vi "ReceiveTCPfromPi_Binary_queue.vi"() -> ()   [LabVIEW 2014]
uses:
  <vilib>/Utility/file.llb/Write To Spreadsheet File (string).vi
  <vilib>/Utility/file.llb/Write To Spreadsheet File (DBL).vi
panel:
  in  "Description":string
  out "Binary File Refnum":refnum<file>
  in  "Record":bool
  in  "Plot 3":u16(ring) items=["gpsTimeUTC", "cT", "EKF VelN", "EKF VelE", "EKF VelD", "EKF PosN", "EKF PosE", "EKF PosD", "EKF Roll", "EKF Pitch", "EKF Yaw", "EKF Lat", "EKF Lon", "EKF Alt", "CMP VelN", "CMP VelE", "CMP VelD", "CMP PosN", "CMP PosE", "CMP PosD", "CMP Roll", "CMP Pitch", "CMP Yaw", "CMP Lat", "CMP Lon", "CMP Alt", "GPS Lat", "GPS Lon", "GPS Alt", "GPS VelN", "GPS VelE", "GPS VelD", "AccelX", "AccelY", "AccelZ", "GyroX", "GyroY", "GyroZ", "MagX", "MagY", "MagZ", "piAlpha", "piPfwd", "piP45", "ardAlpha", "ardPfwd", "ardP45", "Alpha", "Beta"]
  in  "Plot 2":u16(ring) items=["gpsTimeUTC", "cT", "EKF VelN", "EKF VelE", "EKF VelD", "EKF PosN", "EKF PosE", "EKF PosD", "EKF Roll", "EKF Pitch", "EKF Yaw", "EKF Lat", "EKF Lon", "EKF Alt", "CMP VelN", "CMP VelE", "CMP VelD", "CMP PosN", "CMP PosE", "CMP PosD", "CMP Roll", "CMP Pitch", "CMP Yaw", "CMP Lat", "CMP Lon", "CMP Alt", "GPS Lat", "GPS Lon", "GPS Alt", "GPS VelN", "GPS VelE", "GPS VelD", "AccelX", "AccelY", "AccelZ", "GyroX", "GyroY", "GyroZ", "MagX", "MagY", "MagZ", "piAlpha", "piPfwd", "piP45", "ardAlpha", "ardPfwd", "ardP45", "Alpha", "Beta"]
  in  "Plot 1":u16(ring) items=["gpsTimeUTC", "cT", "EKF VelN", "EKF VelE", "EKF VelD", "EKF PosN", "EKF PosE", "EKF PosD", "EKF Roll", "EKF Pitch", "EKF Yaw", "EKF Lat", "EKF Lon", "EKF Alt", "CMP VelN", "CMP VelE", "CMP VelD", "CMP PosN", "CMP PosE", "CMP PosD", "CMP Roll", "CMP Pitch", "CMP Yaw", "CMP Lat", "CMP Lon", "CMP Alt", "GPS Lat", "GPS Lon", "GPS Alt", "GPS VelN", "GPS VelE", "GPS VelD", "AccelX", "AccelY", "AccelZ", "GyroX", "GyroY", "GyroZ", "MagX", "MagY", "MagZ", "piAlpha", "piPfwd", "piP45", "ardAlpha", "ardPfwd", "ardP45", "Alpha", "Beta"]
  out "Num Characters Lost":i32
  out "Spreadsheet Datalog File":path=path "C:/Users/romneyj/Desktop/EKFDatalog2.txt"
  out "Binary Datalog File":path=path "C:/Users/romneyj/Desktop/EKFDatalog.txt"
  out "Chart Values":dbl[](array[numeric]) format="%#_14f"
  out "Chart":cluster{"[0]":dbl, "[1]":dbl, "[2]":dbl}(graph)
  in  "Values to Display":dbl(slide)=100.0 min=10.0 max=2000.0 step=10.0 scale=10.0..2000.0
  out "error out":errorcluster
  out "before substring":string
  in  "stop":bool
  in  "Port":u16=5005
  in  "IP Address":string="155.31.242.65"
  # "Plot Values"
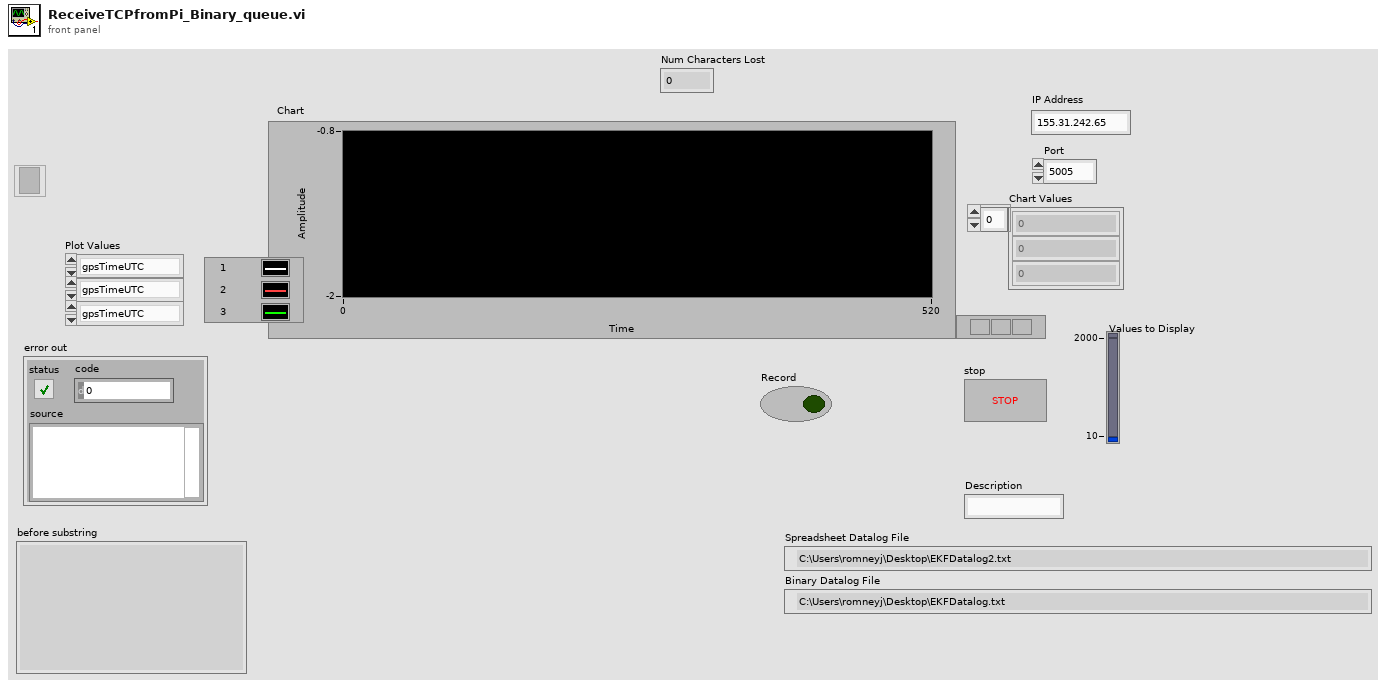
[diagram p1: front panel]
types:
  T1 = cluster{"gpsTimeUTC":i64, "cT":dbl, "EKF VelN":sgl, "EKF VelE":sgl, "EKF VelD":sgl, "EKF PosN":sgl, "EKF PosE":sgl, "EKF PosD":sgl, "EKF Roll":sgl, "EKF Pitch":sgl, "EKF Yaw":sgl, "EKF Lat":dbl, "EKF Lon":dbl, "EKF Alt":sgl, "CMP VelN":sgl, "CMP VelE":sgl, "CMP VelD":sgl, "CMP PosN":sgl, "CMP PosE":sgl, "CMP PosD":sgl, "CMP Roll":sgl, "CMP Pitch":sgl, "CMP Yaw":sgl, "CMP Lat":dbl, "CMP Lon":dbl, "CMP Alt":sgl, "GPS Lat":dbl, "GPS Lon":dbl, "GPS Alt":sgl, "GPS VelN":sgl, "GPS VelE":sgl, "GPS VelD":sgl, "AccelX":sgl, "AccelY":sgl, "AccelZ":sgl, "GyroX":sgl, "GyroY":sgl, "GyroZ":sgl, "MagX":sgl, "MagY":sgl, "MagZ":sgl, "piAlpha":sgl, "piPfwd":u16, "piP45":u16, "ardAlpha":sgl, "ardPfwd":u16, "ardP45":u16, "Alpha":sgl, "Beta":sgl}
  T2 = enum16{"open", "replace", "create", "open or create", "replace or create", "replace or create with confirmation"}
  T3 = enum16{"big-endian, network order", "native, host order", "little-endian"}
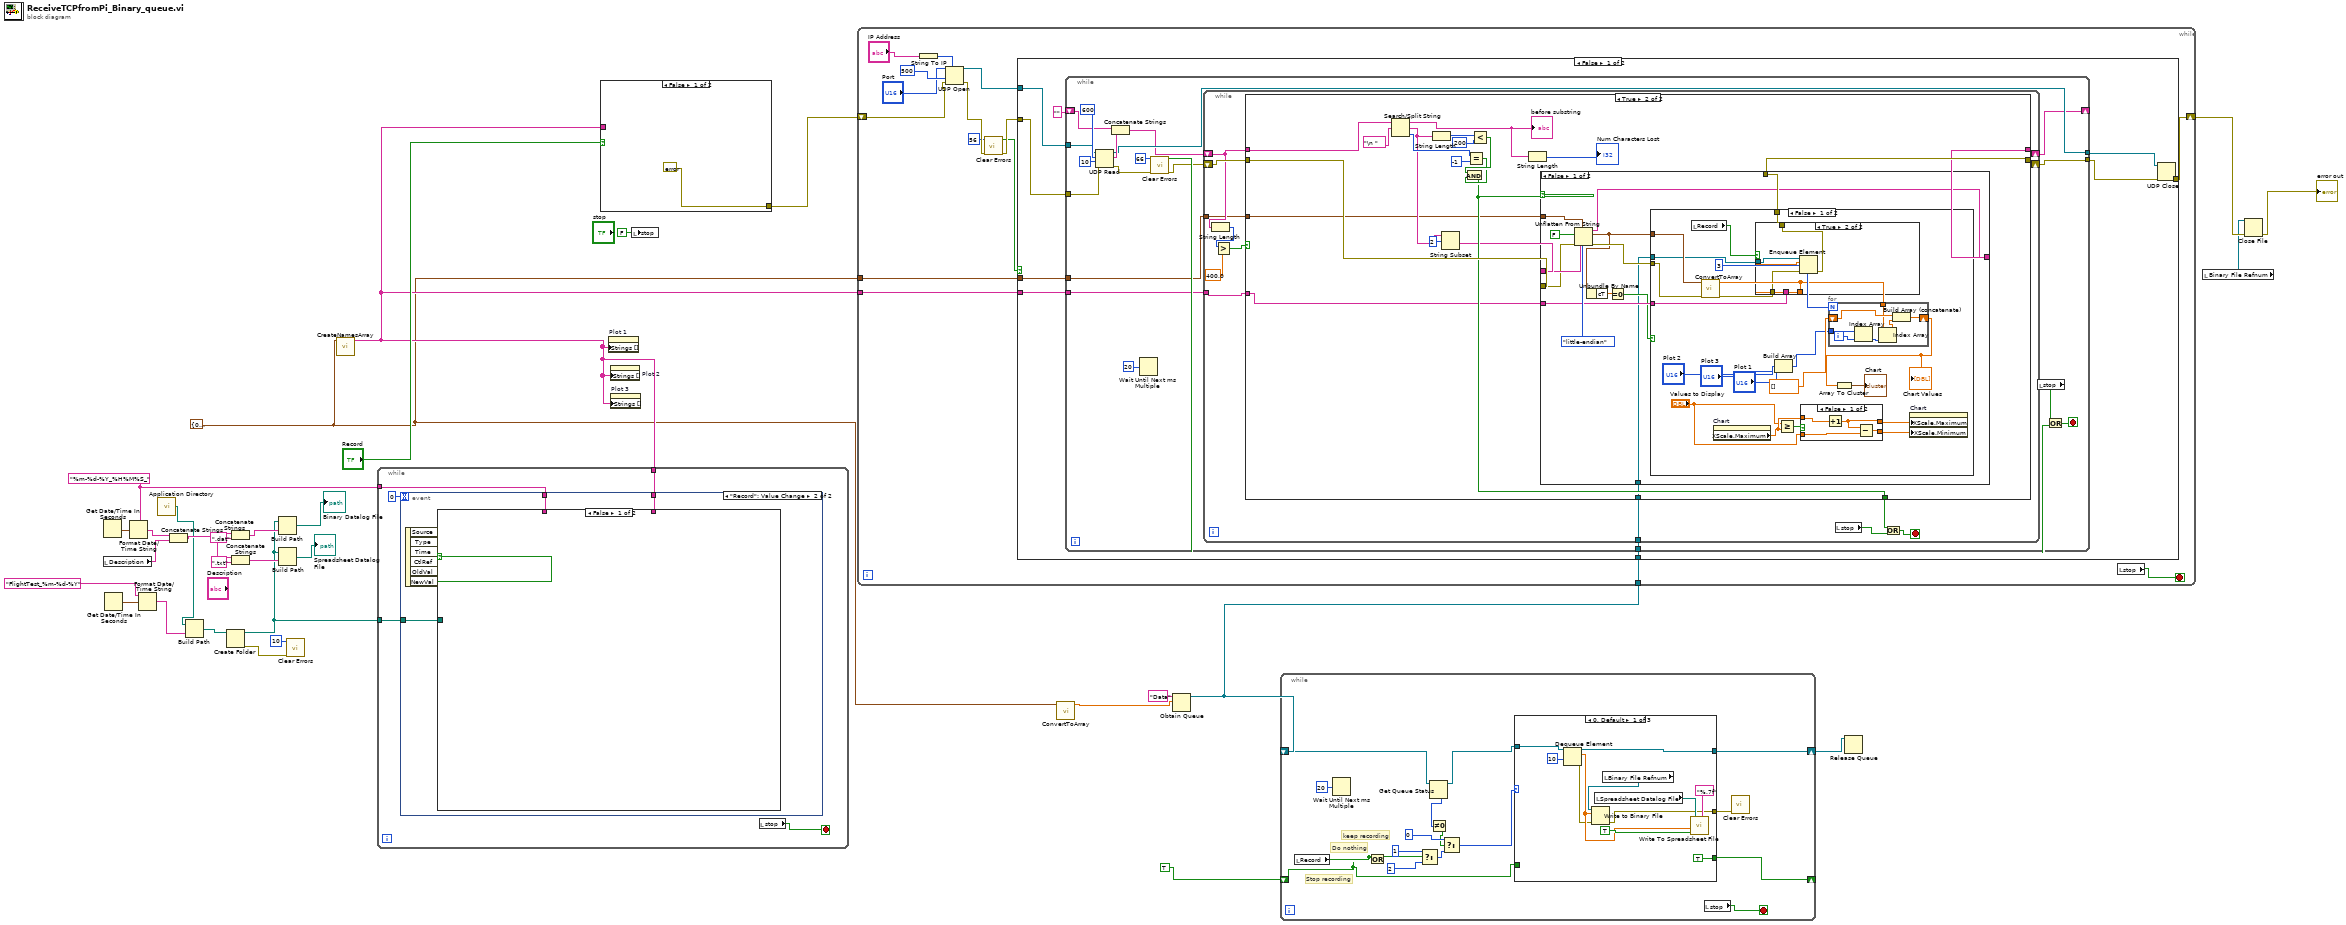
[diagram p0: block diagram]
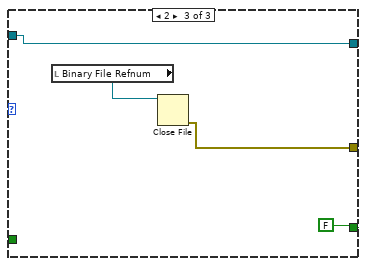
[diagram p3: hidden frame]
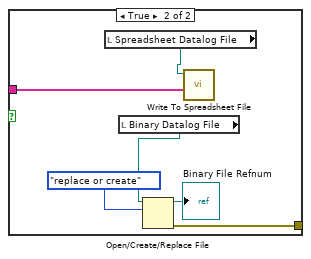
[diagram p4: hidden frame]
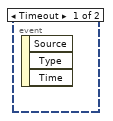
[diagram p5: hidden frame]
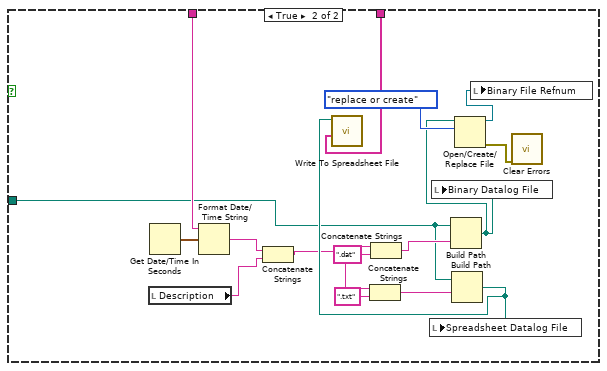
[diagram p6: hidden frame]
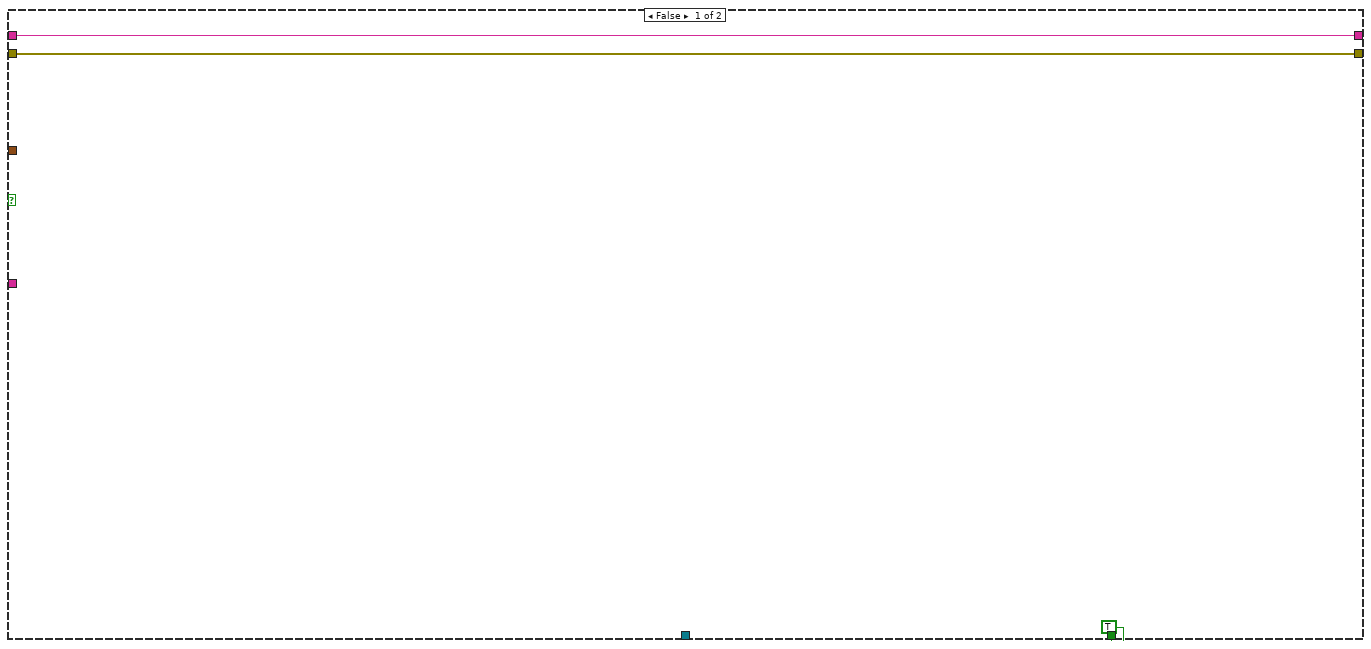
[diagram p7: hidden frame]
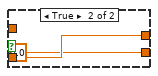
[diagram p9: hidden frame]
diagram:
  w18 = "%m-%d-%Y_%H%M%S_" ("time format string (%c)")
  w3 = T1 {"gpsTimeUTC"=0, "cT"=0.0, "EKF VelN"=0.0, "EKF VelE"=0.0, "EKF VelD"=0.0, "EKF PosN"=0.0, "EKF PosE"=0.0, "EKF PosD"=0.0, "EKF Roll"=0.0, "EKF Pitch"=0.0, "EKF Yaw"=0.0, "EKF Lat"=0.0, "EKF Lon"=0.0, "EKF Alt"=0.0, "CMP VelN"=0.0, "CMP VelE"=0.0, "CMP VelD"=0.0, "CMP PosN"=0.0, "CMP PosE"=0.0, "CMP PosD"=0.0, "CMP Roll"=0.0, "CMP Pitch"=0.0, "CMP Yaw"=0.0, "CMP Lat"=0.0, "CMP Lon"=0.0, "CMP Alt"=0.0, "GPS Lat"=0.0, "GPS Lon"=0.0, "GPS Alt"=0.0, "GPS VelN"=0.0, "GPS VelE"=0.0, "GPS VelD"=0.0, "AccelX"=0.0, "AccelY"=0.0, "AccelZ"=0.0, "GyroX"=0.0, "GyroY"=0.0, "GyroZ"=0.0, "MagX"=0.0, "MagY"=0.0, "MagZ"=0.0, "piAlpha"=0.0, "piPfwd"=0, "piP45"=0, "ardAlpha"=0.0, "ardPfwd"=0, "ardP45"=0, "Alpha"=0.0, "Beta"=0.0}
  n1 = local read "Description"() -> (w17:string)
  n2 = Get Date/Time In Seconds() -> (seconds since 1Jan1904=w19:timestamp)
  n3 = Get Date/Time In Seconds() -> (seconds since 1Jan1904=w14:timestamp)
  n4 = Format Date/Time String(time format string (%c)=w18, seconds (now)=w19) -> (date/time string=w16:string)  [unwired: 1 in]
  n5 = Format Date/Time String(time format string (%c)="FlightTest_%m-%d-%Y", seconds (now)=w14) -> (date/time string=w13:string)  [unwired: 1 in]
  n6 = call <vilib>:"Application Directory.vi"() -> ("Application Directory"=w12:path)
  n7 = Concatenate Strings(w16, w17) -> (w26:string)
  n8 = Build Path(base path=w12, name or relative path=w13) -> (appended path=w11:path)
  n9 = Create Folder(path (use dialog)=w11) -> (created path=w10:path, error out=w9:errorcluster)  [unwired: 2 in, 1 out]
  n10 = Concatenate Strings(w26, ".txt" ("string")) -> (w24:string)
  n11 = Concatenate Strings(w26, ".dat" ("string")) -> (w25:string)
  n12 = Build Path(base path=w10, name or relative path=w25) -> (appended path=→"Binary Datalog File":path)
  n13 = Build Path(base path=w10, name or relative path=w24) -> (appended path=→"Spreadsheet Datalog File":path)
  n14 = call <vilib>:"Clear Errors.vi"("error in (no error)"=w9, "specific error code to clear (0: all)"=10) -> ()  [unwired: 4 in, 2 out]
  n15 = call "CreateNamesArray.vi"("Cluster"=w3) -> ("Array"=w7:string[])  [unwired: 10 in]
  n16 = while {
    tunnel: w7 -> [w36]
    tunnel: w18 -> [w34]
    tunnel: w10 -> [w33]
    stop <- w37 stop-if-true
    n17 = event shown="[1] \"Record\": Value Change" {
      selector: _ -> [_ _]
      dyn-events: _ -> [_ _]
      timeout: 0 -> [_ _]
      tunnel: w36 -> [_ w40]
      tunnel: w34 -> [_ w39]
      tunnel: w33 -> [_ w38]
      event Timeout {
        n18 = event-data() -> ()  [unwired: 1 in, 3 out]
      }
      event "Record": Value Change {
        n19 = event-data() -> ("NewVal"=w41:bool)  [unwired: 1 in, 5 out]
        n20 = case shown="False" w41 {
          tunnel: w40 -> [_ w57]
          tunnel: w39 -> [_ w46]
          tunnel: w38 -> [_ w42]
          frame False {
          }
          frame True {
            n21 = local read "Description"() -> (w43:string)
            n22 = Get Date/Time In Seconds() -> (seconds since 1Jan1904=w45:timestamp)
            n23 = Format Date/Time String(time format string (%c)=w46, seconds (now)=w45) -> (date/time string=w44:string)  [unwired: 1 in]
            n24 = Concatenate Strings(w44, w43) -> (w47:string)
            n25 = Concatenate Strings(w47, ".txt" ("string")) -> (w51:string)
            n26 = Concatenate Strings(w47, ".dat" ("string")) -> (w50:string)
            n27 = Build Path(base path=w42, name or relative path=w50) -> (appended path=w49:path)
            n28 = local write "Binary Datalog File"(w49) -> ()
            n29 = Build Path(base path=w42, name or relative path=w51) -> (appended path=w48:path)
            n30 = call-poly <vilib>:"Write To Spreadsheet File.vi"("1D data"=w57, "file path (dialog if empty)"=w48) -> ()  [unwired: 6 in, 1 out]
            n31 = local write "Spreadsheet Datalog File"(w48) -> ()
            n32 = Open/Create/Replace File(file path (use dialog)=w49, operation (0:open)=T2."replace or create") -> (refnum out=w56:refnum<file>, error out=w55:errorcluster)  [unwired: 4 in, 1 out]
            n33 = local write "Binary File Refnum"(w56) -> ()
            n34 = call <vilib>:"Clear Errors.vi"("error in (no error)"=w55) -> ()  [unwired: 5 in, 2 out]
          }
        }
      }
    }
    n35 = local read "stop"() -> (w37:bool)
  }
  n36 = case shown="False" "Record" {
    tunnel: [errorcluster {"status"=FALSE, "code"=0, "source"=""} ("error out") w63] -> w29
    tunnel: w7 -> [_ w61]
    frame False {
    }
    frame True {
      n37 = local read "Spreadsheet Datalog File"() -> (w62:path)
      n38 = local read "Binary Datalog File"() -> (w59:path)
      n39 = Open/Create/Replace File(file path (use dialog)=w59, operation (0:open)=T2."replace or create") -> (refnum out=→"Binary File Refnum":refnum<file>, error out=w63:errorcluster)  [unwired: 4 in, 1 out]
      n40 = call-poly <vilib>:"Write To Spreadsheet File.vi"("1D data"=w61, "file path (dialog if empty)"=w62) -> ()  [unwired: 6 in, 1 out]
    }
  }
  n41 = property on="Plot 1" class="Ring (strict)"("Strings []"=w7) -> ()  [unwired: 2 in, 2 out]
  n42 = property on="Plot 2" class="Ring (strict)"("Strings []"=w7) -> ()  [unwired: 2 in, 2 out]
  n43 = property on="Plot 3" class="Ring (strict)"("Strings []"=w7) -> ()  [unwired: 2 in, 2 out]
  n44 = local write "stop"(FALSE ("stop")) -> ()
  n45 = call "ConvertToArray.vi"("Cluster"=w3) -> ("Array"=w4:dbl[])  [unwired: 9 in, 1 out]
  n46 = Obtain Queue(name (unnamed)="Data", element data type=w4) -> (queue out=w1:refnum<queue>)  [unwired: 3 in, 2 out]
  n47 = while {
    shift-right: [w75] -> w31
    shift-left: w29 -> [w76]
    tunnel: w3 -> [w68]
    tunnel: w7 -> [w67]
    tunnel: w1 -> [w65]
    stop <- w74 stop-if-true
    n48 = String To IP(1:"IP Address") -> (0:w78:u32)
    n49 = UDP Open(7:w78, 8:w76, 9:500 ("timeout ms (wait forever: -1)"), 11:"Port") -> (port=w77:refnum<k16>, 0:w72:errorcluster)  [unwired: 1 in, 1 out]
    n50 = call <vilib>:"Clear Errors.vi"("error in (no error)"=w72, "specific error code to clear (0: all)"=56) -> ("error out"=w71:errorcluster, "specific error cleared?"=w69:bool)  [unwired: 4 in]
    n51 = case shown="False" w69 {
      tunnel: w77 -> [w88 _]
      tunnel: [w85 w200] -> w75
      tunnel: w71 -> [w84 w200]
      tunnel: w68 -> [w83 _]
      tunnel: w67 -> [w82 _]
      tunnel: w65 -> [w80 _]
      frame False {
        n52 = while {
          tunnel: w88 -> [w90]
          tunnel: w84 -> [w105]
          shift-right: [w101] -> _
          shift-left: "" -> [w104]
          tunnel: [w103] -> w81
          tunnel: [w102] -> w86
          tunnel: w83 -> [w93]
          tunnel: w82 -> [w92]
          tunnel: w80 -> [w89]
          stop <- w96 stop-if-true
          n53 = UDP Read(connection ID=w90, max size (548)=600 ("bytes to read"), timeout ms (25000)=10, 8:w105) -> (data out=w108:string, error out=w95:errorcluster, 3:w103:refnum<k16>)  [unwired: 2 out]
          n54 = Concatenate Strings(w104, w108) -> (w100:string)
          n55 = Wait Until Next ms Multiple(millisecond multiple=u32 20) -> ()  [unwired: 1 out]
          n56 = call <vilib>:"Clear Errors.vi"("error in (no error)"=w95, "specific error code to clear (0: all)"=66 ("error code (no error:0)")) -> ("error out"=w94:errorcluster, "specific error cleared?"=w97:bool)  [unwired: 4 in]
          n57 = while {
            shift-right: [w120] -> w102
            shift-left: w94 -> [w121]
            shift-right: [w119] -> w101
            shift-left: w100 -> [w112]
            tunnel: w93 -> [w111]
            tunnel: w92 -> [w110]
            tunnel: w89 -> [w109]
            stop <- w115 stop-if-true
            n58 = String Length(string=w112) -> (length=w117:i32)
            n59 = Greater?(x=w117, y=400.0) -> (0:w116:bool)
            n60 = case shown="True" w116 {
              tunnel: w121 -> [w123 w134]
              tunnel: w112 -> [w124 w142]
              tunnel: [w123 w144] -> w120
              tunnel: [w124 w135] -> w119
              tunnel: [TRUE w133] -> w113
              tunnel: w111 -> [_ w127]
              tunnel: w110 -> [_ w126]
              tunnel: w109 -> [_ w125]
              frame False {
              }
              frame True {
                n61 = Search/Split String(string=w142, search string/char (-)="\n " ("regular expression")) -> (substring before match=w132:string, match + rest of string=w130:string, offset of match=w141:i32)  [unwired: 1 in]
                "before substring" <- w132
                n62 = String Length(string=w130) -> (length=w139:i32)
                n63 = String Subset(string=w130, offset (0)=2) -> (substring=w129:string)  [unwired: 1 in]
                n64 = Equal?(x=w141, y=-1) -> (x = y?=w136:bool)
                n65 = Less?(x=w139, y=200) -> (x < y?=w137:bool)
                n66 = And(x=w137, y=w136) -> (x .and. y?=w133:bool)
                n67 = String Length(string=w132) -> (length=→"Num Characters Lost":i32)
                n68 = case shown="False" w133 {
                  tunnel: [w157 w199] -> w144
                  tunnel: [w154 w198] -> w135
                  tunnel: w129 -> [w153 w198]
                  tunnel: w134 -> [w152 w199]
                  tunnel: w127 -> [w148 _]
                  tunnel: w126 -> [w147 _]
                  tunnel: w125 -> [w145 _]
                  frame False {
                    n69 = Unflatten From String(type=w148, binary string=w153, data includes array or string size? (T)=FALSE, byte order (0:big-endian, network order)=T3."little-endian", error in (no error)=w152) -> (rest of the binary string=w154:string, value=w150:T1, error out=w155:errorcluster)
                    n70 = Unbundle By Name(w150) -> ("cT"=w149:dbl)
                    n71 = Equal To 0?(x=w149) -> (x = 0?=w146:bool)
                    n72 = case shown="False" w146 {
                      tunnel: [w178 w197] -> w157
                      tunnel: w155 -> [w164 w197]
                      tunnel: w150 -> [w162 _]
                      tunnel: w147 -> [w160 _]
                      tunnel: w145 -> [w158 _]
                      frame False {
                        n73 = local read "Record"() -> (w159:bool)
                        n74 = call "ConvertToArray.vi"("error in (no error)"=w164, "Cluster"=w162) -> ("error out"=w163:errorcluster, "Array"=w161:dbl[])  [unwired: 8 in]
                        n75 = property on="Chart" class="WFChart (strict)"() -> ("XScale.Maximum"=w173:dbl)  [unwired: 2 in, 2 out]
                        n76 = case shown="True" w159 {
                          tunnel: [w179 w182] -> w178
                          tunnel: w163 -> [w179 w183]
                          tunnel: w161 -> [_ w181]
                          tunnel: w160 -> [_ _]
                          tunnel: w158 -> [_ w180]
                          frame False {
                          }
                          frame True {
                            n77 = Enqueue Element(queue=w180, element=w181, error in (no error)=w183) -> (error out=w182:errorcluster)  [unwired: 1 in, 2 out]
                          }
                        }
                        n78 = Build Array("Plot 1", "Plot 2", "Plot 3") -> (w168:u16[])
                        n79 = Greater Or Equal?(x="Values to Display", y=w173) -> (x >= y?=w169:bool)
                        n80 = case shown="False" w169 {
                          tunnel: "Values to Display" -> [w186 w189]
                          tunnel: [w185 w189] -> w171
                          tunnel: [w187 0.0] -> w172
                          tunnel: w173 -> [w184 _]
                          frame False {
                            n81 = Increment(x=w184) -> (x+1=w185:dbl)
                            n82 = Subtract(x=w185, y=w186) -> (x-y=w187:dbl)
                          }
                          frame True {
                          }
                        }
                        n83 = for {
                          N: 3 ("Number of Plots") -> [_]
                          tunnel: w168 -> [w195]
                          shift-right: [w190] -> w176
                          shift-left: dbl[] [] -> [w194]
                          tunnel: w161 -> [w192]
                          i -> [w193]
                          n84 = Index Array(array=w195, index=w193) -> (element=w196:u16)
                          n85 = Index Array(array=w192, index=w196) -> (element=w191:dbl)
                          n86 = Build Array (concatenate)(w194, w191) -> (w190:dbl[])
                        }
                        "Chart Values" <- w176
                        n87 = Array To Cluster(array=w176) -> (cluster=→"Chart":cluster{"[0]":dbl, "[1]":dbl, "[2]":dbl})
                        n88 = property on="Chart" class="WFChart (strict)"("XScale.Maximum"=w171, "XScale.Minimum"=w172) -> ()  [unwired: 2 in, 2 out]
                      }
                      frame True {
                      }
                    }
                  }
                  frame True {
                  }
                }
              }
            }
            n89 = local read "stop"() -> (w114:bool)
            n90 = Or(x=w113, y=w114) -> (x .or. y?=w115:bool)
          }
          n91 = local read "stop"() -> (w98:bool)
          n92 = Or(x=w98, y=w97) -> (x .or. y?=w96:bool)
        }
        n93 = UDP Close(connection ID=w81, 8:w86) -> (error out=w85:errorcluster)  [unwired: 1 out]
      }
      frame True {
      }
    }
    n94 = local read "stop"() -> (w74:bool)
  }
  n95 = while {
    shift-right: [w215] -> w5
    shift-left: w1 -> [w208]
    shift-right: [w204] -> _
    shift-left: TRUE -> [w203]
    stop <- w216 stop-if-true
    # "keep recording"
    # "Do nothing"
    # "Stop recording"
    n96 = local read "Record"() -> (w205:bool)
    n97 = Wait Until Next ms Multiple(millisecond multiple=u32 20) -> ()  [unwired: 1 out]
    n98 = Or(x=w205, y=w203) -> ()  [unwired: 1 out]
    n99 = Select(t=1, s=w205, f=2) -> (s? t:f=w209:i32)
    n100 = Get Queue Status(queue=w208) -> (queue out=w207:refnum<queue>, # elements in queue=w214:i32)  [unwired: 2 in, 6 out]
    n101 = Not Equal To 0?(x=w214) -> (x != 0?=w210:bool)
    n102 = Select(t=0, s=w210, f=w209) -> (s? t:f=w206:i32)
    n103 = case shown="0, Default" w206 {
      tunnel: w207 -> [w227 w229 w233]
      tunnel: [w226 w229 w233] -> w215
      tunnel: [TRUE w228 FALSE] -> w204
      tunnel: w203 -> [_ w228 _]
      tunnel: [w218 _ w230] -> w201
      frame 0, Default {
        n104 = Dequeue Element(queue=w227, timeout in ms (-1)=10) -> (queue out=w226:refnum<queue>, element=w219:dbl[], error out=w217:errorcluster)  [unwired: 1 in, 1 out]
        n105 = local read "Spreadsheet Datalog File"() -> (w222:path)
        n106 = local read "Binary File Refnum"() -> (w223:refnum<file>)
        n107 = Write to Binary File(file (use dialog)=w223, data=w219, error in=w217) -> (error out=w218:errorcluster)  [unwired: 3 in, 2 out]
        n108 = call-poly <vilib>:"Write To Spreadsheet File.vi"("format (%.3f)"="%.7f", "append to file? (new file:F)"=TRUE, "1D data"=w219, "file path (dialog if empty)"=w222) -> ()  [unwired: 4 in, 1 out]
      }
      frame 1 {
      }
      frame 2 {
        n109 = local read "Binary File Refnum"() -> (w231:refnum<file>)
        n110 = Close File(refnum=w231) -> (error out=w230:errorcluster)  [unwired: 1 in, 1 out]
      }
    }
    n111 = local read "stop"() -> (w216:bool)
    n112 = call <vilib>:"Clear Errors.vi"("error in (no error)"=w201) -> ()  [unwired: 5 in, 2 out]
  }
  n113 = Release Queue(queue=w5) -> ()  [unwired: 2 in, 3 out]
  n114 = local read "Binary File Refnum"() -> (w28:refnum<file>)
  n115 = Close File(refnum=w28, error in=w31) -> (error out=→"error out":errorcluster)  [unwired: 1 out]
